vi "Helium3 Pressure to Temperature.vi"(11 "He3 Pressure (mbar)":dbl=0.4 format="%_5e") -> (3 "He3 Temperature (K)":dbl format="%_6f")   [LabVIEW 2020]
uses:
  <vilib>/Analysis/polynomials.llb/Scalar Polynomial Evaluation (DBL).vi
  <vilib>/Analysis/NI_AALPro.lvlib
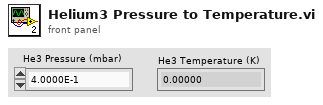
[diagram p1: front panel]
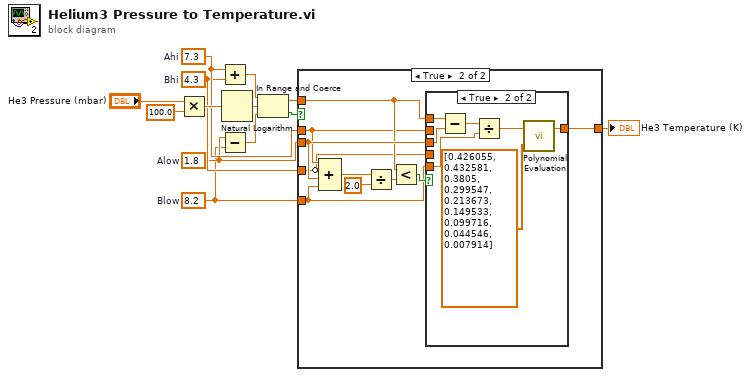
[diagram p0: block diagram]
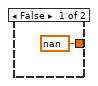
[diagram p2: hidden frame]
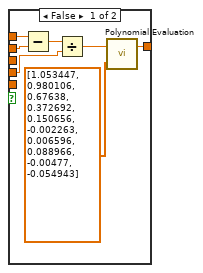
[diagram p3: hidden frame]
diagram:
  w3 = 4.3  # Bhi
  w4 = 7.3  # Ahi
  w1 = 8.2  # Blow
  w2 = 1.8  # Alow
  n1 = Multiply(x="He3 Pressure (mbar)", y=100.0) -> (x*y=w11:dbl)
  n2 = Add(x=w4, y=w3) -> (x+y=w9:dbl)
  n3 = Subtract(x=w2, y=w1) -> (x-y=w10:dbl)
  n4 = Natural Logarithm(1:w11) -> (0:w8:dbl)
  n5 = In Range and Coerce(upper limit=w9, x=w8, lower limit=w10) -> (coerced(x)=w6:dbl, In Range?=w7:bool)
  n6 = case shown="True" w7 {
    tunnel: w6 -> [_ w19]
    tunnel: [nan w17] -> w5
    tunnel: w4 -> [_ w16]
    tunnel: w3 -> [_ w15]
    tunnel: w2 -> [_ w20]
    tunnel: w1 -> [_ w18]
    frame False {
    }
    frame True {
      n7 = Compound Arithmetic op=unknown(w16, invert w15, w20, w18) -> (w24:dbl)
      n8 = Divide(x=w24, y=2.0) -> (x/y=w22:dbl)
      n9 = Less?(x=w19, y=w22) -> (x < y?=w21:bool)
      n10 = case shown="True" w21 {
        tunnel: w20 -> [_ w38]
        tunnel: w19 -> [w27 w37]
        tunnel: w18 -> [_ w35]
        tunnel: [w28 w32] -> w17
        tunnel: w16 -> [w26 _]
        tunnel: w15 -> [w25 _]
        frame False {
          n11 = Subtract(x=w27, y=w26) -> (x-y=w31:dbl)
          n12 = Divide(x=w31, y=w25) -> (x/y=w29:dbl)
          n13 = call-poly <vilib>:"Polynomial Evaluation.vi"("P(x)"=dbl[] [1.053447, 0.980106, 0.67638, 0.372692, 0.150656, -0.002263, 0.006596, 0.088966, -0.00477, -0.054943], "a"=w29) -> ("P(a)"=w28:dbl)  [unwired: 1 out]
        }
        frame True {
          n14 = Subtract(x=w37, y=w38) -> (x-y=w36:dbl)
          n15 = Divide(x=w36, y=w35) -> (x/y=w33:dbl)
          n16 = call-poly <vilib>:"Polynomial Evaluation.vi"("P(x)"=dbl[] [0.426055, 0.432581, 0.3805, 0.299547, 0.213673, 0.149533, 0.099716, 0.044546, 0.007914], "a"=w33) -> ("P(a)"=w32:dbl)  [unwired: 1 out]
        }
      }
    }
  }
  "He3 Temperature (K)" <- w5
